vi "Add Multiple.vi"(0 "Assembly in":refnum<class "Assembly Run.lvclass">, 1 "Settings":T1, 3 "Position":i32, 7 "Modules":refnum<class "Module.lvclass">[](array[class]), 11 "error in (no error)":errorcluster, 12 "Baseplate Tray ID":i32, 13 "Component Tray ID":i32, 14 "Glue step":enum16{"Kapton", "Sensor", "PCB"}(ring)) -> (4 "Assembly out":refnum<class "Assembly Run.lvclass">, 15 "error out":errorcluster)   [LabVIEW 2016, in "Assembly Run.lvclass"]
uses:
  Assembly Run.lvclass
  Routine/Settings.ctl
  Routine/Routine.lvclass
  Module/Module.lvclass
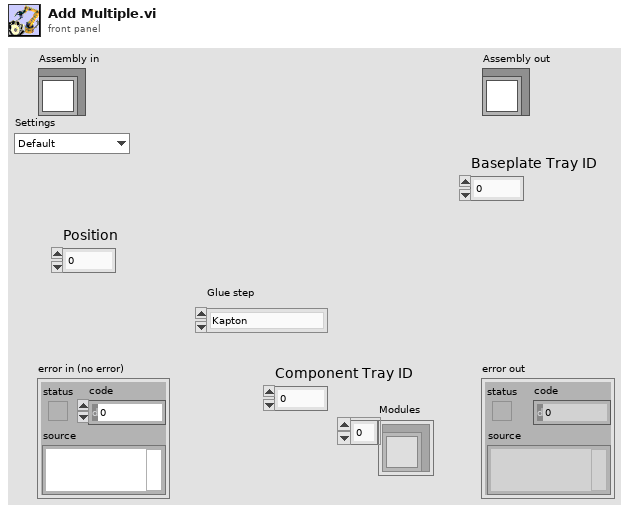
[diagram p1: front panel]
types:
  T1 = typedef "Routine.lvclass/Settings.ctl" = enum16{"Default", "Custom"}
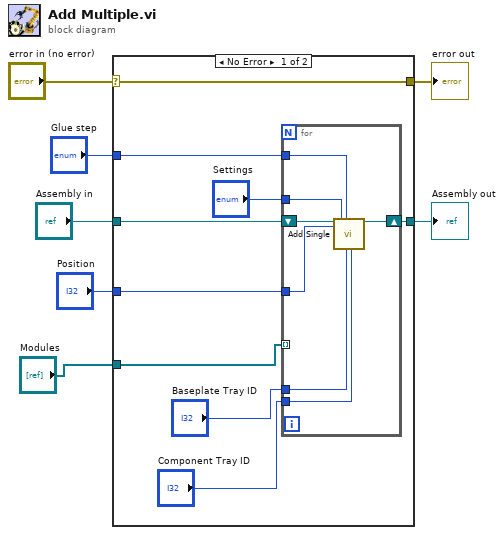
[diagram p0: block diagram]
diagram:
  n1 = case shown="No Error" "error in (no error)" {
    selector: "error in (no error)" -> [w16 w25]
    tunnel: [w16 w25] -> w6
    tunnel: [w14 w24] -> w4
    tunnel: "Assembly in" -> [w15 w24]
    tunnel: "Position" -> [w10 _]
    tunnel: "Glue step" -> [w9 _]
    tunnel: "Modules" -> [w8 _]
    frame No Error {
      n2 = for {
        shift-right: [w21] -> w14
        shift-left: w15 -> [w23]
        tunnel: "Settings" -> [w22]
        tunnel: "Baseplate Tray ID" -> [w20]
        tunnel: "Component Tray ID" -> [w19]
        tunnel: w10 -> [w18]
        tunnel: w9 -> [w17]
        tunnel: w8 -> [_] mode=indexing
        n3 = call-dynamic "Add Single.vi"("UI in"=w23, "position"=w18, "Settings"=w22, "Glue step"=w17, "Baseplate Tray ID"=w20, "Component Tray ID"=w19) -> ("UI out"=w21:refnum<class "Assembly Run.lvclass">)  [unwired: 12 in, 1 out]
      }
    }
    frame Error {
    }
  }
  "error out" <- w6
  "Assembly out" <- w4
